vi "Stop Heater.vi"(8 "error in (no error)":errorcluster, 11 "Freezer in":refnum<class "Freezer.lvclass">) -> (0 "error out":errorcluster, 3 "Freezer out":refnum<class "Freezer.lvclass">)   [LabVIEW 2015, in "cRIO-Carbondioxide.lvlib" / "CO2-Actor.lvlib" / "Freezer.lvclass"]
uses:
  Freezer.lvclass
  Freezer.lvclass/Freezer.ctl
  <vilib>/ActorFramework/Message Enqueuer/Message Enqueuer.lvclass/Message Enqueuer.ctl
  <vilib>/ActorFramework/Message Enqueuer/Enqueue.vi
  <vilib>/ActorFramework/Message Priority Queue/Priority Enqueue.vi
  <vilib>/ActorFramework/Stop Msg/Stop Msg.lvclass
  CO2 Actor/CO2 Actor.lvclass
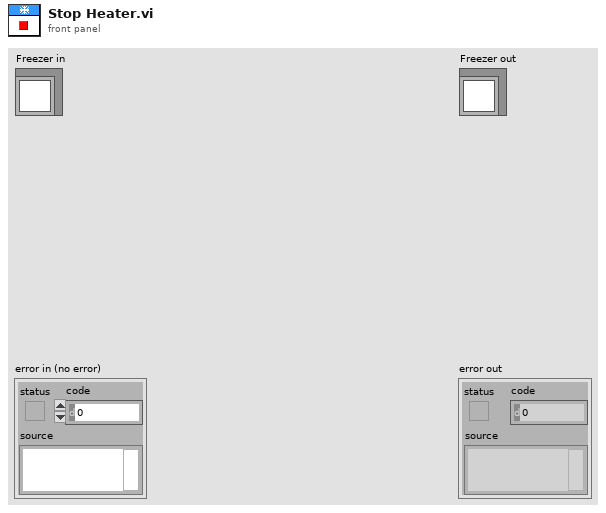
[diagram p1: front panel]
types:
  T1 = typedef "cRIO-Carbondioxide.lvlib/cRIO-CO2.lvlib/cRIO-CO2.lvclass/Blowers Heaters Enumerator.ctl" = enum16{"Tank Blower 1", "Tank Blower 2", "Tank Blower 3", "Tank Blower 4", "Syringe Blower", "Syringe Heater", "Piston Heater", "Undefined"}
  T2 = typedef "Dedicated Enqueuers.ctl" = cluster{"Freezers":cluster{"Syringe":refnum<class "Message Enqueuer.lvclass">, "Tank 1":refnum<class "Message Enqueuer.lvclass">, "Tank 2":refnum<class "Message Enqueuer.lvclass">, "Tank 3":refnum<class "Message Enqueuer.lvclass">, "Tank 4":refnum<class "Message Enqueuer.lvclass">}, "Heaters":cluster{"Syringe":refnum<class "Message Enqueuer.lvclass">, "Piston":refnum<class "Message Enqueuer.lvclass">}, "Blowers":cluster{"Tank 1":refnum<class "Message Enqueuer.lvclass">, "Tank 2":refnum<class "Message Enqueuer.lvclass">, "Tank 3":refnum<class "Message Enqueuer.lvclass">, "Tank 4":refnum<class "Message Enqueuer.lvclass">, "Syringe":refnum<class "Message Enqueuer.lvclass">}, "Sample Line":refnum<class "Message Enqueuer.lvclass">, "Storage Line":refnum<class "Message Enqueuer.lvclass">, "Transfer Line":refnum<class "Message Enqueuer.lvclass">, "Syringe Stepper":refnum<class "Message Enqueuer.lvclass">, "Syringe Line":refnum<class "Message Enqueuer.lvclass">, "Capillary Line":refnum<class "Message Enqueuer.lvclass">, "Preparation Line":refnum<class "Message Enqueuer.lvclass">, "Turbo":refnum<class "Message Enqueuer.lvclass">, "Vacuum":refnum<class "Message Enqueuer.lvclass">, "He Line":refnum<class "Message Enqueuer.lvclass">, "Cylinder":refnum<class "Message Enqueuer.lvclass">}
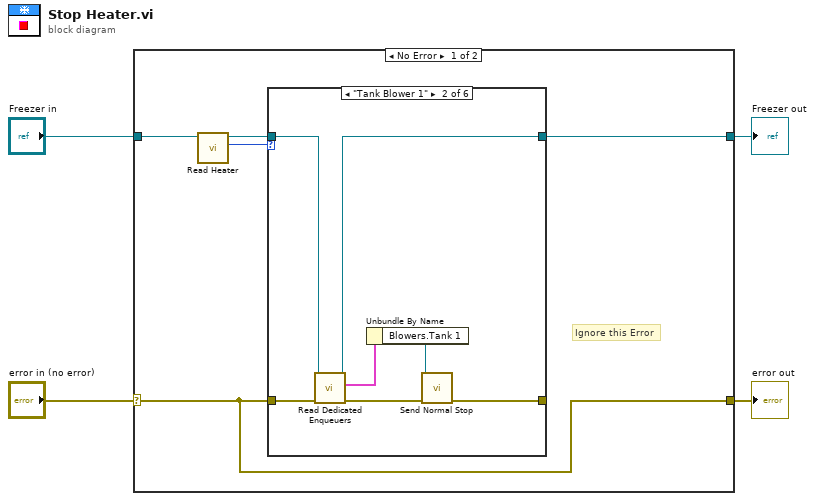
[diagram p0: block diagram]
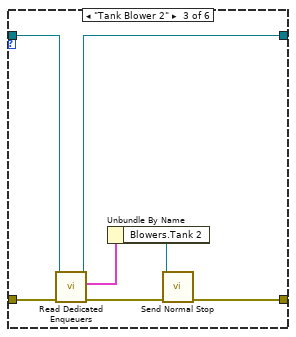
[diagram p3: hidden frame]
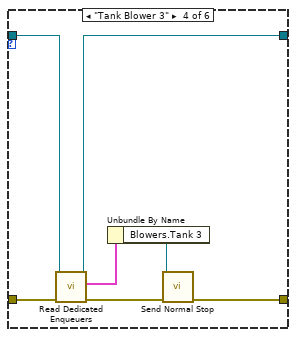
[diagram p4: hidden frame]
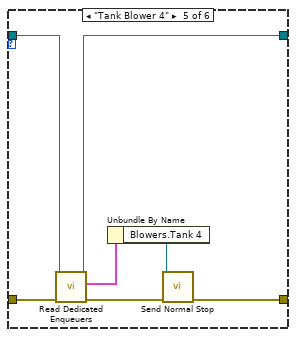
[diagram p5: hidden frame]
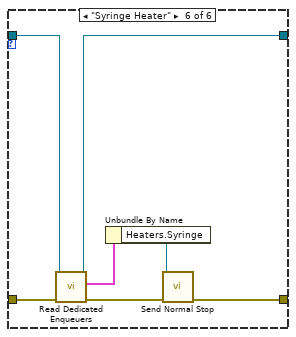
[diagram p6: hidden frame]
diagram:
  n1 = case shown="No Error" "error in (no error)" {
    selector: "error in (no error)" -> [w5 w48]
    tunnel: [w5 w48] -> w3
    tunnel: [w7 w47] -> w1
    tunnel: "Freezer in" -> [w9 w47]
    frame No Error {
      # "Ignore this Error"
      n2 = call "Read Heater.vi"("Freezer in"=w9) -> ("Blower/Heater"=w6:T1, "Freezer out"=w8:refnum<class "Freezer.lvclass">)  [unwired: 9 in]
      n3 = case shown="\"Tank Blower 1\"" w6 {
        tunnel: w5 -> [w10 w18 w25 w32 w39 w46]
        tunnel: [w10 w13 w20 w27 w34 w40] -> _
        tunnel: w8 -> [w11 w17 w24 w31 w38 w45]
        tunnel: [w11 w16 w23 w30 w37 w44] -> w7
        frame "Undefined", Default {
        }
        frame "Tank Blower 1" {
          n4 = call "Read Dedicated Enqueuers.vi"("error in (no error)"=w18, "CO2 Actor in"=w17) -> ("error out"=w14:errorcluster, "Dedicated Enqueuers"=w15:T2, "CO2 Actor out"=w16:refnum<class "Freezer.lvclass">)  [unwired: 6 in, 1 out]
          n5 = Unbundle By Name(w15) -> ("Blowers.Tank 1"=w12:refnum<class "Message Enqueuer.lvclass">)
          n6 = call <vilib>:"Send Normal Stop.vi"("error in (no error)"=w14, "Message Enqueuer"=w12) -> ("error out"=w13:errorcluster)  [unwired: 9 in]
        }
        frame "Tank Blower 2" {
          n7 = call "Read Dedicated Enqueuers.vi"("error in (no error)"=w25, "CO2 Actor in"=w24) -> ("error out"=w21:errorcluster, "Dedicated Enqueuers"=w22:T2, "CO2 Actor out"=w23:refnum<class "Freezer.lvclass">)  [unwired: 6 in, 1 out]
          n8 = Unbundle By Name(w22) -> ("Blowers.Tank 2"=w19:refnum<class "Message Enqueuer.lvclass">)
          n9 = call <vilib>:"Send Normal Stop.vi"("error in (no error)"=w21, "Message Enqueuer"=w19) -> ("error out"=w20:errorcluster)  [unwired: 9 in]
        }
        frame "Tank Blower 3" {
          n10 = call "Read Dedicated Enqueuers.vi"("error in (no error)"=w32, "CO2 Actor in"=w31) -> ("error out"=w28:errorcluster, "Dedicated Enqueuers"=w29:T2, "CO2 Actor out"=w30:refnum<class "Freezer.lvclass">)  [unwired: 6 in, 1 out]
          n11 = Unbundle By Name(w29) -> ("Blowers.Tank 3"=w26:refnum<class "Message Enqueuer.lvclass">)
          n12 = call <vilib>:"Send Normal Stop.vi"("error in (no error)"=w28, "Message Enqueuer"=w26) -> ("error out"=w27:errorcluster)  [unwired: 9 in]
        }
        frame "Tank Blower 4" {
          n13 = call "Read Dedicated Enqueuers.vi"("error in (no error)"=w39, "CO2 Actor in"=w38) -> ("error out"=w35:errorcluster, "Dedicated Enqueuers"=w36:T2, "CO2 Actor out"=w37:refnum<class "Freezer.lvclass">)  [unwired: 6 in, 1 out]
          n14 = Unbundle By Name(w36) -> ("Blowers.Tank 4"=w33:refnum<class "Message Enqueuer.lvclass">)
          n15 = call <vilib>:"Send Normal Stop.vi"("error in (no error)"=w35, "Message Enqueuer"=w33) -> ("error out"=w34:errorcluster)  [unwired: 9 in]
        }
        frame "Syringe Heater" {
          n16 = call "Read Dedicated Enqueuers.vi"("error in (no error)"=w46, "CO2 Actor in"=w45) -> ("error out"=w41:errorcluster, "Dedicated Enqueuers"=w43:T2, "CO2 Actor out"=w44:refnum<class "Freezer.lvclass">)  [unwired: 6 in, 1 out]
          n17 = Unbundle By Name(w43) -> ("Heaters.Syringe"=w42:refnum<class "Message Enqueuer.lvclass">)
          n18 = call <vilib>:"Send Normal Stop.vi"("error in (no error)"=w41, "Message Enqueuer"=w42) -> ("error out"=w40:errorcluster)  [unwired: 9 in]
        }
      }
    }
    frame Error {
    }
  }
  "error out" <- w3
  "Freezer out" <- w1
